vi "Configure Limit Test Lower Limit.vi"(0 "VISA resource name":refnum<visa-resource-name>, 5 "Limit Test Number (1)":u16=1, 7 "Lower Limit (-1.0)":dbl=-1.0, 9 "Function (0: Volts)":u16(ring) items=["Volts", "Current", "Resistance", "Digitize Voltage", "Digitize Current"], 11 "error in (no error)":errorcluster) -> (4 "VISA resource name out":refnum<visa-resource-name>, 15 "error out":errorcluster)   [LabVIEW 2021, in "Keithley 2450.lvlib"]
doc: "This sets the lower limit of the limit test."
uses:
  <instrlib>/Keithley 2450/Keithley 2450.lvlib
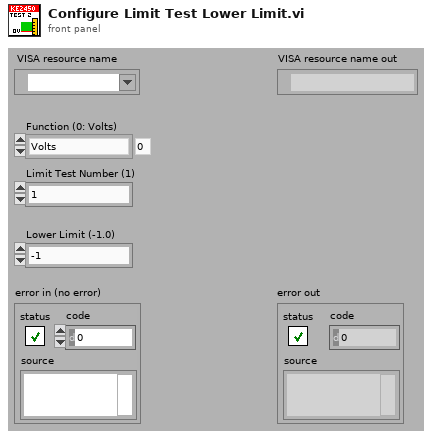
[diagram p1: front panel]
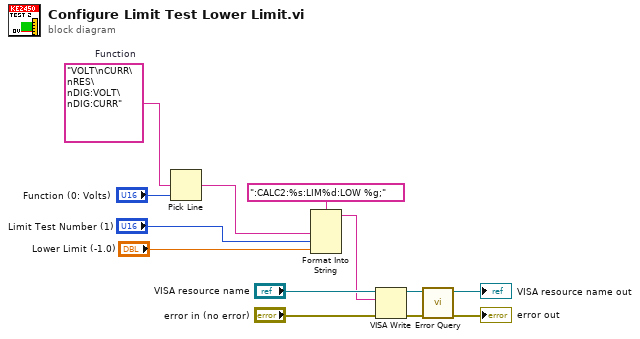
[diagram p0: block diagram]
diagram:
  w5 = "VOLT\nCURR\nRES\nDIG:VOLT\nDIG:CURR"  # Function
  n1 = Pick Line(multi-line string=w5, line index="Function (0: Volts)") -> (output string=w3:string)  [unwired: 1 out]
  n2 = Format Into String(format string=":CALC2:%s:LIM%d:LOW %g;", w3, "Limit Test Number (1)", "Lower Limit (-1.0)") -> (resulting string=w6:string)  [unwired: 2 in, 1 out]
  n3 = VISA Write(VISA resource name="VISA resource name", write buffer=w6, error in (no error)="error in (no error)") -> (VISA resource name out=w9:refnum<visa-resource-name>, error out=w8:errorcluster)  [unwired: 1 out]
  n4 = call <instrlib>:"Error Query.vi"("error in (no error)"=w8, "VISA resource name"=w9) -> ("error out"=→"error out":errorcluster, "VISA resource name out"=→"VISA resource name out":refnum<visa-resource-name>)  [unwired: 8 out]
